vi "OE_Product_selection_list.vi"(7 "Numeric":i32, 8 "error in (no error)":errorcluster, 9 "Plan data":string[][](array[string])) -> (0 "error out":errorcluster, 2 "Disabled":T1(ring), 3 "Array out":T2(array[cluster]))   [LabVIEW 2017]
uses:
  <userlib>/_OpenG.lib/array/array.llb/Remove Duplicates from 1D Array (String)__ogtk.vi
panel:
  out "array":string[](array[string])
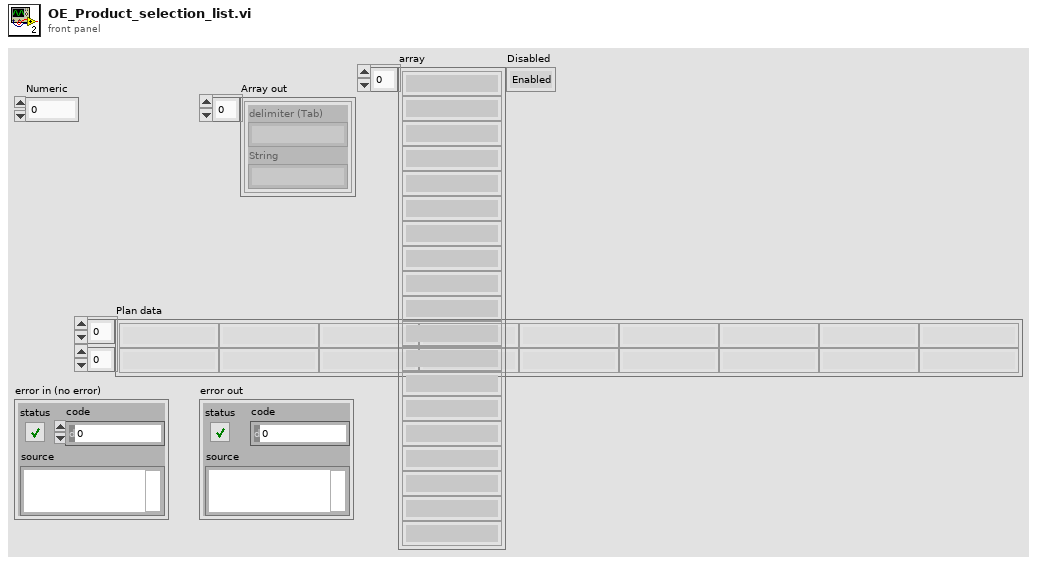
[diagram p1: front panel]
types:
  T1 = enum8{"Enabled", "Disabled", "Disabled and Grayed Out"}
  T2 = cluster{"delimiter (Tab)":string, "String":string}[]
  T3 = enum32{"invalid app kind", "Development System", "Run Time System", "Student Edition", "Embedded LabVIEW", "Evaluation", "Custom"}
  T4 = cluster{"delimiter (Tab)":string, "String":string}
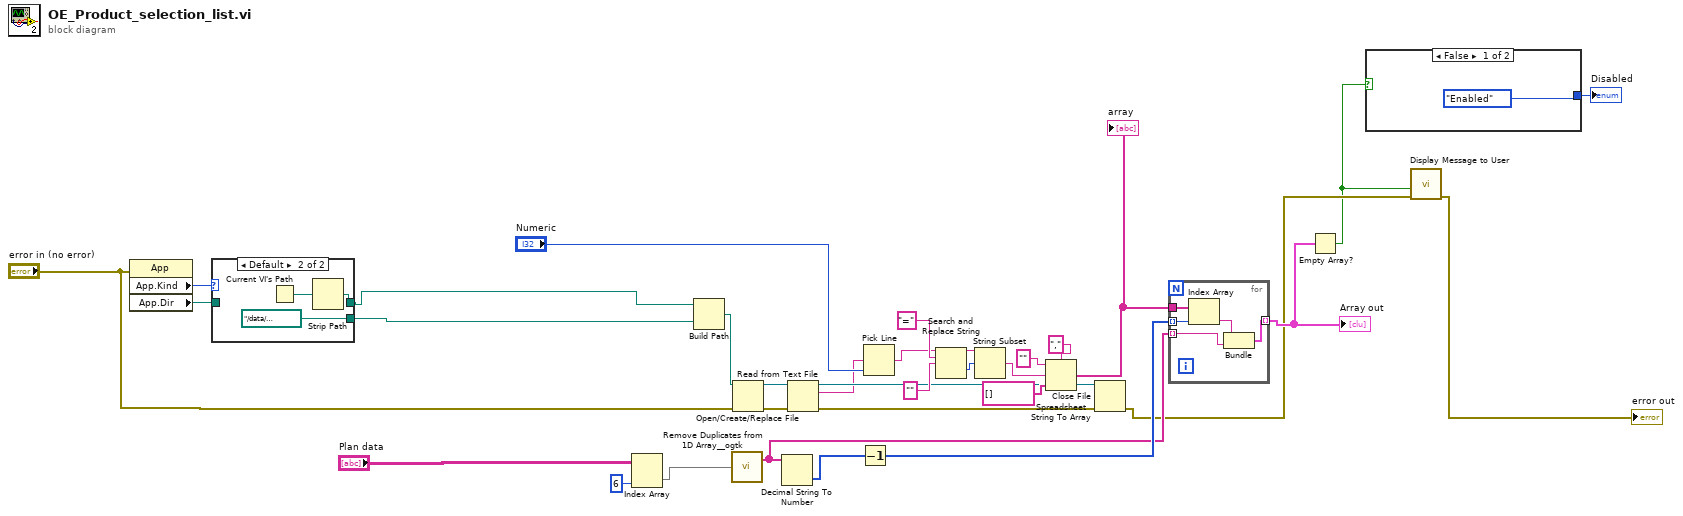
[diagram p0: block diagram]
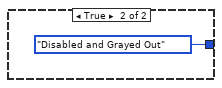
[diagram p2: hidden frame]
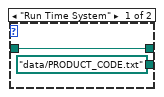
[diagram p3: hidden frame]
diagram:
  n1 = property class="App"(error in="error in (no error)") -> ("App.Kind"=w10:T3, "App.Dir"=w11:path)  [unwired: 1 in, 2 out]
  n2 = case shown="Default" w10 {
    tunnel: w11 -> [w35 _]
    tunnel: [path "data/PRODUCT_CODE.txt" ("path") path "../data/PRODUCT_CODE.txt" ("path")] -> w9
    tunnel: [w35 w36] -> w8
    frame "Run Time System" {
    }
    frame Default {
      n3 = Current VI's Path() -> (path=w37:path)
      n4 = Strip Path(path=w37) -> (stripped path=w36:path)  [unwired: 1 out]
    }
  }
  n5 = Index Array(array="Plan data", index (col)=6 ("disabled index (col)")) -> (element=w13:string[])  [unwired: 1 in]
  n6 = Build Path(base path=w8, name or relative path=w9) -> (appended path=w26:path)
  n7 = call-poly <userlib>:"Remove Duplicates from 1D Array__ogtk.vi"("Input Array"=w13) -> ("Output Array"=w6:string[])  [unwired: 1 out]
  n8 = Open/Create/Replace File(file path (use dialog)=w26, error in="error in (no error)") -> (refnum out=w25:refnum<file>, error out=w24:errorcluster)  [unwired: 4 in, 1 out]
  n9 = Decimal String To Number(string=w6) -> (number=w15:i32[])  [unwired: 2 in, 1 out]
  n10 = Read from Text File(file (use dialog)=w25, error in=w24) -> (refnum out=w22:refnum<file>, text=w21:string, error out=w23:errorcluster)  [unwired: 2 in, 1 out]
  n11 = Decrement(x=w15) -> (x-1=w14:i32[])
  n12 = Pick Line(multi-line string=w21, line index="Numeric") -> (output string=w17:string)  [unwired: 1 in]
  n13 = Search and Replace String(input string=w17, search string="=" ("format string"), replace string="" ("search string")) -> (result string=w19:string, offset past replacement=w20:i32)  [unwired: 5 in, 2 out]
  n14 = String Subset(string=w19, offset (0)=w20) -> (substring=w18:string)  [unwired: 1 in]
  n15 = Spreadsheet String To Array(delimiter (Tab)=",", format string="", spreadsheet string=w18, array type (2D Dbl)=string[] [] ("delimiter (Tab)")) -> (array=w33:string[])
  "array" <- w33
  n16 = Close File(refnum=w22, error in=w23) -> (error out=w4:errorcluster)  [unwired: 1 out]
  n17 = for {
    tunnel: w14 -> [w43] mode=indexing
    tunnel: w33 -> [w42]
    tunnel: [w39] -> w5 mode=indexing
    tunnel: w6 -> [w41] mode=indexing
    n18 = Index Array(array=w42, index=w43) -> (element=w40:string)
    n19 = Bundle("delimiter (Tab)"=w40, "String"=w41) -> (w39:T4)  [unwired: 1 in]
  }
  "Array out" <- w5
  n20 = Empty Array?(array=w5) -> (empty?=w2:bool)
  n21 = case shown="False" w2 {
    tunnel: [T1."Enabled" ("Disabled") T1."Disabled and Grayed Out" ("Disabled")] -> w1
    frame False {
    }
    frame True {
    }
  }
  "Disabled" <- w1
  n22 = call "Display Message to User"("error in (no error)"=w4, "Enable"=w2) -> ("error out"=→"error out":errorcluster)  [unwired: 8 in, 1 out]
